vi "MGI Create Logger.vi"(8 "error in (no error)":errorcluster, 9 "Ignore Warnings? (F: Process Errors and Warnings)":bool, 10 "Error Log Directory \n(Not a Path: Shared Docs\\Caller Prefix)\n(\"\" Path: Turn off logging)":path=path "", 11 "Error Reporter":refnum<class "MGI Error Reporter Base.lvclass">) -> (0 "error out":errorcluster, 2 "Error Log Directory Used":path, 3 "Already Running?":bool)   [LabVIEW 2020, in "MGI Error Reporter Base.lvclass"]
doc: "Starts an Error Reporter daemon using the optionally wired Error Reporter. If Error Reporter is not wired, then the default behavior is used, which is to log errors but not display a window.\nIf an Error Reporter daemon is already running from a top level VI, do nothing and output True for \"Already Running\". See \"VI Tree.vi\" for more details.\n\nAuthored by Shawn Walpole\nsupport@mooregoodideas.com\nwww.mooregoodideas.com\n\nCopyright (c) 2013, Moore Good Ideas, Inc.\n\nAll rights reserved.\n\nRedistribution and use in source and binary forms, with or without modification, are permitted provided that the following conditions are met:\n\n * Redistributions of source code must retain the above copyright notice, this list of conditions and the following disclaimer.\n * Redistributions in binary form must reproduce the above copyright notice, this list of conditions and the following disclaimer in the documentation and/or other materials provided with the distribution.\n * Neither the name of Moore Good Ideas, Inc. nor the names of its contributors may be used to endorse or promote products derived from this software without specific prior written permission.\n\nTHIS SOFTWARE IS PROVIDED BY THE COPYRIGHT HOLDERS AND CONTRIBUTORS \"AS IS\" AND ANY EXPRESS OR IMPLIED WARRANTIES, INCLUDING, BUT NOT LIMITED TO, THE IMPLIED WARRANTIES OF MERCHANTABILITY AND FITNESS FOR A PARTICULAR PURPOSE ARE DISCLAIMED. IN NO EVENT SHALL THE COPYRIGHT OWNER OR CONTRIBUTORS BE LIABLE FOR ANY DIRECT, INDIRECT, INCIDENTAL, SPECIAL, EXEMPLARY, OR CONSEQUENTIAL DAMAGES (INCLUDING, BUT NOT LIMITED TO, PROCUREMENT OF SUBSTITUTE GOODS OR SERVICES; LOSS OF USE, DATA, OR PROFITS; OR BUSINESS INTERRUPTION) HOWEVER CAUSED AND ON ANY THEORY OF LIABILITY, WHETHER IN CONTRACT, STRICT LIABILITY, OR TORT (INCLUDING NEGLIGENCE OR OTHERWISE) ARISING IN ANY WAY OUT OF THE USE OF THIS SOFTWARE, EVEN IF ADVISED OF THE POSSIBILITY OF SUCH DAMAGE."
uses:
  <userlib>/_MGI/Error Reporter/MGI Error Reporter Base/MGI Error Reporter Base.lvclass
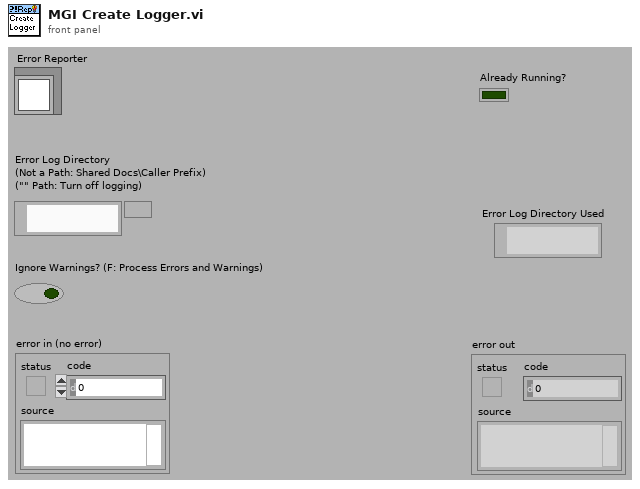
[diagram p1: front panel]
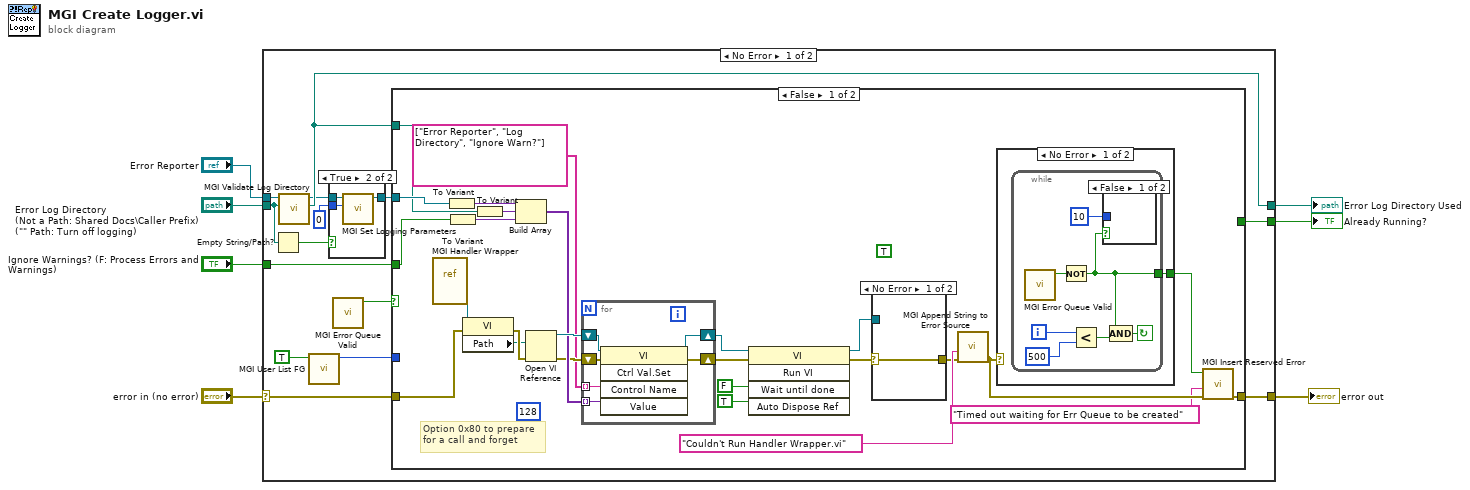
[diagram p0: block diagram]
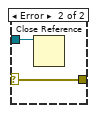
[diagram p3: hidden frame]
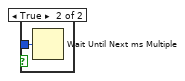
[diagram p4: hidden frame]
diagram:
  n1 = case shown="No Error" "error in (no error)" {
    selector: "error in (no error)" -> [w20 w73]
    tunnel: "Error Reporter" -> [w18 _]
    tunnel: [w19 w73] -> w6
    tunnel: "Error Log Directory \n(Not a Path: Shared Docs\\Caller Prefix)\n(\"\" Path: Turn off logging)" -> [w16 w72]
    tunnel: [w14 w72] -> w4
    tunnel: [w10 _] -> w3
    tunnel: "Ignore Warnings? (F: Process Errors and Warnings)" -> [w9 _]
    frame No Error {
      n2 = Empty String/Path?(string/path=w16) -> (empty?=w15:bool)
      n3 = call-dynamic "MGI Validate Log Directory.vi"("Log Directory (<Not a Path>: Use Default)"=w16, "MGI Error Reporter In"=w18) -> ("Validated Path"=w14:path, "MGI Error Reporter Out"=w13:refnum<class "MGI Error Reporter Base.lvclass">)  [unwired: 8 out]
      n4 = call <userlib>:"MGI User List FG.vi"("Create? (F:Destroy)"=TRUE) -> ("# Top Level Users"=w17:i32)  [unwired: 10 out]
      n5 = case shown="True" w15 {
        tunnel: w13 -> [w22 w25]
        tunnel: [w22 w24] -> w12
        tunnel: 0 ("Max # Errors to Log (Don't change)") -> [_ w23]
        frame False {
        }
        frame True {
          n6 = call <userlib>:"MGI Set Logging Parameters.vi"("Max # Errors to Log (Don't change)"=w23, "MGI Error Reporter Base In"=w25) -> ("MGI Error Reporter Base Out"=w24:refnum<class "MGI Error Reporter Base.lvclass">)  [unwired: 9 out]
        }
      }
      n7 = call <userlib>:"MGI Error Queue Valid.vi"() -> ("Error Queue Valid?"=w8:bool)  [unwired: 11 out]
      n8 = case shown="False" w8 {
        selector: w8 -> [_ w70]
        tunnel: w12 -> [w40 _]
        tunnel: [w48 w71] -> w19
        tunnel: w20 -> [w43 w71]
        tunnel: w14 -> [w38 _]
        tunnel: w17 -> [_ _]
        tunnel: [_ w70] -> w10
        tunnel: w9 -> [w36 _]
        frame False {
          (unwired) 128 ("options")
          (unwired) TRUE ("Wait Until Done")
          # "Option 0x80 to prepare\nfor a call and forget"
          n9 = vi-ref <userlib>:"MGI Handler Wrapper.vi"() -> (w44:refnum<vi>)
          n10 = To Variant(anything=w40) -> (Variant=w39:variant)
          n11 = To Variant(anything=w36) -> (Variant=w35:variant)
          n12 = property class="VI"(reference=w44, error in=w43) -> (error out=w46:errorcluster, "Path"=w45:path)  [unwired: 1 out]
          n13 = To Variant(anything=w38) -> (Variant=w37:variant)
          n14 = Build Array(w39, w37, w35) -> (w34:variant[])
          n15 = Open VI Reference(vi path=w45, error in (no error)=w46) -> (vi reference=w41:refnum<vi>, error out=w33:errorcluster)  [unwired: 4 in]
          n16 = for {
            tunnel: w34 -> [w59] mode=indexing
            shift-right: [w58] -> w29
            shift-left: w33 -> [w57]
            tunnel: string[] ["Error Reporter", "Log Directory", "Ignore Warn?"] -> [w56] mode=indexing
            shift-right: [w55] -> w28
            shift-left: w41 -> [w60]
            n17 = invoke class="VI" method="Ctrl Val.Set"(reference=w60, error in=w57, "Control Name"=w56, "Value"=w59) -> (reference out=w55:refnum<vi>, error out=w58:errorcluster)  [unwired: 1 in, 3 out]
          }
          n18 = invoke class="VI" method="Run VI"(reference=w28, error in=w29, "Wait until done"=FALSE ("Wait Until Done"), "Auto Dispose Ref"=TRUE ("Auto Dispose Reference")) -> (reference out=w27:refnum<vi>, error out=w26:errorcluster)  [unwired: 1 in, 3 out]
          n19 = case shown="No Error" w26 {
            selector: w26 -> [w52 w53]
            tunnel: [w52 w53] -> w42
            tunnel: w27 -> [_ w54]
            frame No Error {
            }
            frame Error {
              n20 = Close Reference(reference=w54) -> ()  [unwired: 1 in, 1 out]
            }
          }
          n21 = call <userlib>:"MGI Append String to Error Source.vi"("Error In"=w42, "String to Append"="Couldn't Run Handler Wrapper.vi") -> ("Error Out"=w49:errorcluster)  [unwired: 2 in, 7 out]
          n22 = case shown="No Error" w49 {
            tunnel: [w61 _] -> w50
            frame No Error {
              n23 = while {
                tunnel: [w62] -> w61
                i -> [w67]
                stop <- w68 continue-if-true
                n24 = call <userlib>:"MGI Error Queue Valid.vi"() -> ("Error Queue Valid?"=w63:bool)  [unwired: 11 out]
                n25 = Not(x=w63) -> (.not. x?=w62:bool)
                n26 = Less?(x=w67, y=500 ("millisecond multiple")) -> (x < y?=w64:bool)
                n27 = case shown="False" w62 {
                  tunnel: u32 10 ("millisecond multiple") -> [_ w69]
                  frame False {
                  }
                  frame True {
                    n28 = Wait Until Next ms Multiple(millisecond multiple=w69) -> ()  [unwired: 1 out]
                  }
                }
                n29 = Compound Arithmetic op=AND(w62, w64) -> (w68:bool)
              }
            }
            frame Error {
            }
          }
          n30 = call <userlib>:"MGI Insert Reserved Error.vi"("Error In"=w49, "Error Description"="Timed out waiting for Err Queue to be created", "Error? (T)"=w50) -> ("Error Out"=w48:errorcluster)  [unwired: 1 in, 7 out]
        }
        frame True {
        }
      }
    }
    frame Error {
    }
  }
  "error out" <- w6
  "Error Log Directory Used" <- w4
  "Already Running?" <- w3
